vi "High_Voltage_Power_Supply_WriteToCSV.vi"(0 "File Path (.csv)":path, 1 "WriteToCSV (T = write)":bool, 5 "error in (no error)":errorcluster, 6 "CH1 VOLTAGE SET (V)":refnum<vi>, 7 "CH2 VOLTAGE SET (V)":refnum<vi>, 8 "CH1 CURRENT SET (mA)":refnum<vi>, 9 "CH2 CURRENT SET (mA)":refnum<vi>, 10 "CH1 VOLTAGE OUT (V)":refnum<vi>, 11 "CH2 VOLTAGE OUT (V)":refnum<vi>, 12 "CH1 CURRENT OUT (mA)":refnum<vi>, 13 "CH2 CURRENT OUT (mA)":refnum<vi>) -> (19 "error out":errorcluster)   [LabVIEW 2016]
doc: "This VI writes the set and out voltages and currents from the High Voltage Power (HVP) Supply to a CSV file.\n\nNo data is saved when the file path is empty or when the WriteToCSV enable is false.\n\nExample: \n File path = Q:\\test\\test1.csv :\n * If file does not exist: A new file \"test1.csv\" is created\n * If file does exist: Data is appended to the file \"test1.csv\"\n\nBachelor's thesis FIIW EA-ICT:\n * Sven Baerten - sven.baerten@student.uhasselt.be\n * Wouter Falise - wouter.falise@student.uhasselt.be"
uses:
  <vilib>/Utility/file.llb/Write Delimited Spreadsheet (string).vi
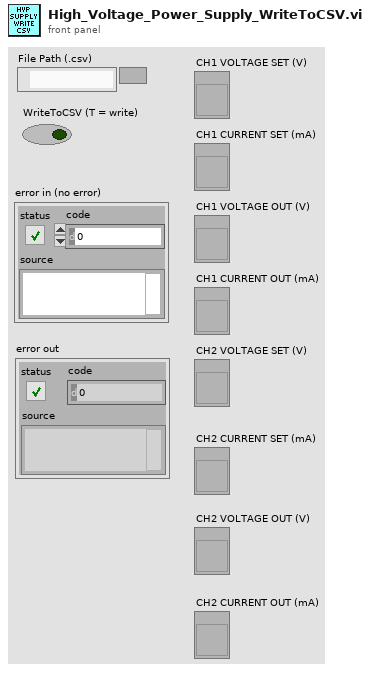
[diagram p1: front panel]
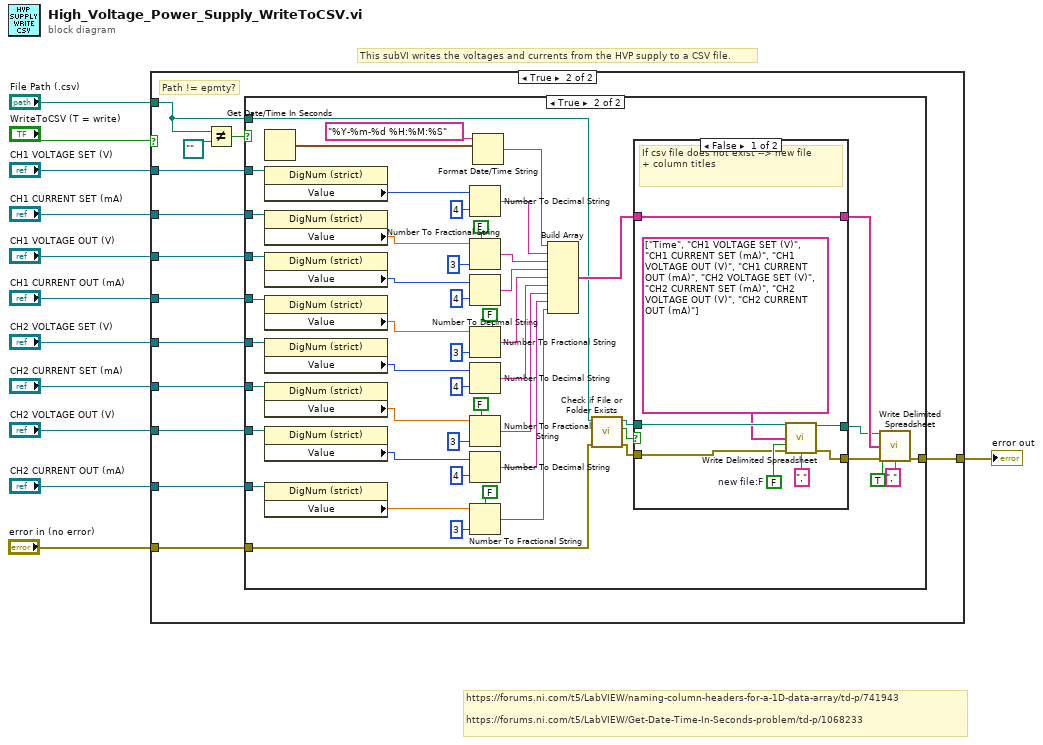
[diagram p0: block diagram]
diagram:
  # "https://forums.ni.com/t5/LabVIEW/naming-column-headers-for-a-1D-data-array/td-p/741943\n\nhttps://forums.ni.com/t5/LabVIEW/Get-Date-Time-In-Seconds-problem/td-p/1068233"
  # "This subVI writes the voltages and currents from the HVP supply to a CSV file."
  n1 = case shown="True" "WriteToCSV (T = write)" {
    tunnel: "File Path (.csv)" -> [_ w16]
    tunnel: "CH1 VOLTAGE SET (V)" -> [_ w24]
    tunnel: "CH1 CURRENT SET (mA)" -> [_ w23]
    tunnel: "CH1 VOLTAGE OUT (V)" -> [_ w22]
    tunnel: "CH2 VOLTAGE SET (V)" -> [_ w21]
    tunnel: "CH2 CURRENT SET (mA)" -> [_ w20]
    tunnel: "CH2 VOLTAGE OUT (V)" -> [_ w19]
    tunnel: "CH2 CURRENT OUT (mA)" -> [_ w18]
    tunnel: "CH1 CURRENT OUT (mA)" -> [_ w17]
    tunnel: "error in (no error)" -> [w13 w15]
    tunnel: [w13 w14] -> w1
    frame False {
    }
    frame True {
      # "Path != epmty?"
      n2 = Not Equal?(x=w16, y=path "") -> (x != y?=w25:bool)
      n3 = case shown="True" w25 {
        tunnel: w16 -> [_ w40]
        tunnel: w24 -> [_ w39]
        tunnel: w23 -> [_ w38]
        tunnel: w22 -> [_ w37]
        tunnel: w21 -> [_ w36]
        tunnel: w20 -> [_ w35]
        tunnel: w19 -> [_ w34]
        tunnel: w18 -> [_ w33]
        tunnel: w17 -> [_ w32]
        tunnel: w15 -> [w27 w31]
        tunnel: [w27 w28] -> w14
        frame False {
        }
        frame True {
          n4 = Get Date/Time In Seconds() -> (seconds since 1Jan1904=w63:timestamp)
          n5 = property on="Property Node" class="DigNum (strict)"(reference=w39) -> ("Value"=w41:i16)  [unwired: 1 in, 2 out]
          n6 = property on="Property Node" class="DigNum (strict)"(reference=w38) -> ("Value"=w42:dbl)  [unwired: 1 in, 2 out]
          n7 = property on="Property Node" class="DigNum (strict)"(reference=w37) -> ("Value"=w43:i32)  [unwired: 1 in, 2 out]
          n8 = property on="Property Node" class="DigNum (strict)"(reference=w32) -> ("Value"=w44:dbl)  [unwired: 1 in, 2 out]
          n9 = property on="Property Node" class="DigNum (strict)"(reference=w36) -> ("Value"=w45:i16)  [unwired: 1 in, 2 out]
          n10 = property on="Property Node" class="DigNum (strict)"(reference=w35) -> ("Value"=w46:dbl)  [unwired: 1 in, 2 out]
          n11 = property on="Property Node" class="DigNum (strict)"(reference=w34) -> ("Value"=w47:i32)  [unwired: 1 in, 2 out]
          n12 = property on="Property Node" class="DigNum (strict)"(reference=w33) -> ("Value"=w48:dbl)  [unwired: 1 in, 2 out]
          n13 = Number To Decimal String(number=w41, width (-)=i16 4) -> (decimal integer string=w53:string)
          n14 = Number To Fractional String(use system decimal point (T)=FALSE, number=w42, precision (6)=i16 3) -> (F-format string=w52:string)  [unwired: 1 in]
          n15 = Number To Decimal String(number=w43, width (-)=i16 4) -> (decimal integer string=w54:string)
          n16 = Number To Fractional String(use system decimal point (T)=FALSE, number=w44, precision (6)=i16 3) -> (F-format string=w55:string)  [unwired: 1 in]
          n17 = Number To Decimal String(number=w45, width (-)=i16 4) -> (decimal integer string=w73:string)
          n18 = Number To Fractional String(use system decimal point (T)=FALSE, number=w46, precision (6)=i16 3) -> (F-format string=w74:string)  [unwired: 1 in]
          n19 = Number To Decimal String(number=w47, width (-)=i16 4) -> (decimal integer string=w75:string)
          n20 = Number To Fractional String(use system decimal point (T)=FALSE, number=w48, precision (6)=i16 3) -> (F-format string=w76:string)  [unwired: 1 in]
          n21 = Format Date/Time String(time format string (%c)="%Y-%m-%d %H:%M:%S", seconds (now)=w63) -> (date/time string=w64:string)  [unwired: 1 in]
          n22 = Build Array(w64, w53, w52, w54, w55, w73, w74, w75, w76) -> (w66:string[])
          n23 = call <vilib>:"Check if File or Folder Exists.vi"("error in (no error)"=w31, "path"=w40) -> ("error out"=w30:errorcluster, "file or folder exists?"=w77:bool, "dup path"=w49:path)  [unwired: 7 in]
          n24 = case shown="False" w77 {
            tunnel: w49 -> [w86 w89]
            tunnel: [w85 w89] -> w50
            tunnel: w66 -> [w81 w88]
            tunnel: [w81 w88] -> w67
            tunnel: w30 -> [w80 w87]
            tunnel: [w79 w87] -> w29
            frame False {
              w84 = FALSE  # new file:F
              # "If csv file does not exist --> new file\n+ column titles"
              n25 = call-poly <vilib>:"Write Delimited Spreadsheet.vi"("file path (dialog if empty)"=w86, "1D data"=string[] ["Time", "CH1 VOLTAGE SET (V)", "CH1 CURRENT SET (mA)", "CH1 VOLTAGE OUT (V)", "CH1 CURRENT OUT (mA)", "CH2 VOLTAGE SET (V)", "CH2 CURRENT SET (mA)", "CH2 VOLTAGE OUT (V)", "CH2 CURRENT OUT (mA)"], "append to file? (new file:F)"=w84, "error in (no error)"=w80, "delimiter (\\t)"="," ("delimiter (\\t)")) -> ("new file path (Not A Path if cancelled)"=w85:path, "error out"=w79:errorcluster)  [unwired: 9 in]
            }
            frame True {
              # "csv file already exists -->\nappend data"
            }
          }
          n26 = call-poly <vilib>:"Write Delimited Spreadsheet.vi"("file path (dialog if empty)"=w50, "1D data"=w67, "append to file? (new file:F)"=TRUE ("append to file:T"), "error in (no error)"=w29, "delimiter (\\t)"="," ("delimiter (\\t)")) -> ("error out"=w28:errorcluster)  [unwired: 9 in, 1 out]
        }
      }
    }
  }
  "error out" <- w1
